vi "update driveble paths (point input).vi"(7 "possible wheel angles":i8[](array[numeric])=[-35, -30, -25, -20, -15, -10, -5, -1, 1, 5, 10, 15, 20, 25, 30, 35], 8 "y LIDAR position(in)":i16, 9 "x LIDAR position(in)":i16, 10 "max path lengths":u16[](array[numeric])=[0, 0, 0, 0, 0, 0, 0, 0, 0, 0, 0, 0, 0, 0, 0, 0], 11 "number 16\" iterations":i32) -> (2 "updated max path lengths":u16[](array[numeric]))   [LabVIEW 2009]
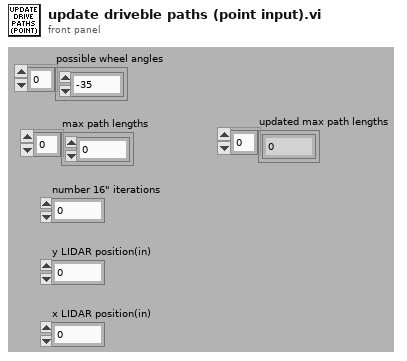
[diagram p1: front panel]
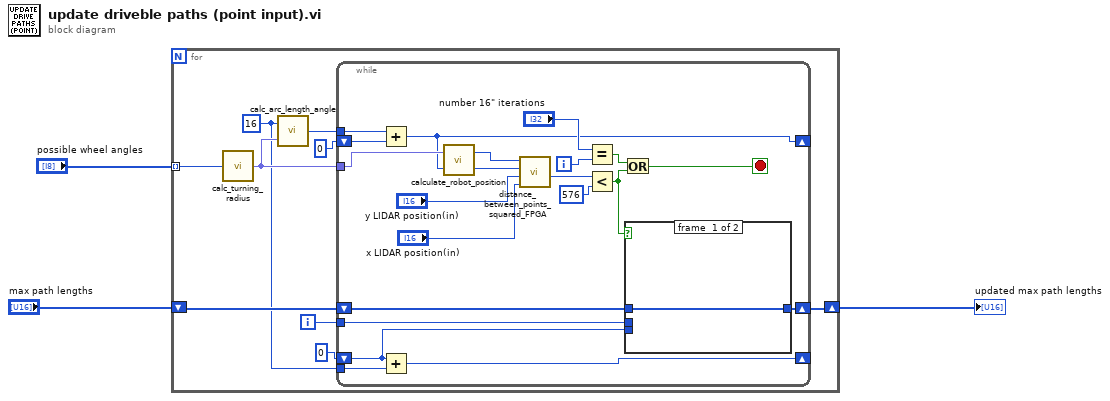
[diagram p0: block diagram]
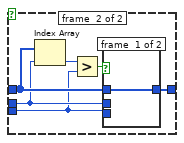
[diagram p2: hidden frame]
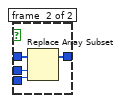
[diagram p3: hidden frame]
diagram:
  n1 = for {
    tunnel: "possible wheel angles" -> [w4] mode=indexing
    shift-right: [w7] -> w1
    shift-left: "max path lengths" -> [w9]
    i -> [w8]
    w6 = u16 16 ("Distance Along Arc")
    n2 = call "calc_turning_radius.vi"("Wheel Angle"=w4) -> ("Turning Radius (in)"=w12:fxp<+/-,22,12>)
    n3 = call "calc_arc_length_angle.vi"("Turning Radius (in)"=w12, "Distance Along Arc"=w6) -> ("arc length angle"=w11:u16)
    n4 = while {
      tunnel: w12 -> [w32]
      tunnel: w11 -> [w33]
      shift-right: [w16] -> _
      shift-left: u16 0 ("arc length angle") -> [w24]
      tunnel: w8 -> [w23]
      shift-right: [w22] -> w7
      shift-left: w9 -> [w25]
      tunnel: w6 -> [w15]
      shift-right: [w14] -> _
      shift-left: u16 0 -> [w13]
      i -> [w21]
      stop <- w17 stop-if-true
      n5 = Add(x=w33, y=w24) -> (x+y=w16:u16)
      n6 = Add(x=w13, y=w15) -> (x+y=w14:u16)
      n7 = call "calculate_robot_position.vi"("arc length angle"=w16, "Turning Radius (in)"=w32) -> ("New Y Position"=w30:i16, "New X Position"=w31:i16)
      n8 = call "distance_between_points_squared_FPGA.vi"("x LIDAR position"="x LIDAR position(in)", "y LIDAR position"="y LIDAR position(in)", "y position"=w30, "x position"=w31) -> ("distance squared"=w27:i32)  [unwired: 7 in]
      n9 = Equal?(x="number 16\" iterations", y=w21) -> (x = y?=w18:bool)
      n10 = Less?(x=w27, y=576) -> (x < y?=w19:bool)
      n11 = Or(x=w18, y=w19) -> (x .or. y?=w17:bool)
      n12 = case shown="True" w19 {
        tunnel: w25 -> [w34 w39]
        tunnel: w13 -> [_ w36]
        tunnel: w23 -> [_ w38]
        tunnel: [w34 w40] -> w22
        frame #0 {
        }
        frame #1 {
          n13 = Index Array(array=w39, index=w38) -> (element=w37:u16)
          n14 = Greater?(x=w37, y=w36) -> (0:w35:bool)
          n15 = case shown="False" w35 {
            tunnel: [w41 w45] -> w40
            tunnel: w39 -> [w41 w44]
            tunnel: w38 -> [_ w43]
            tunnel: w36 -> [_ w42]
            frame #0 {
            }
            frame #1 {
              n16 = Replace Array Subset(array=w44, new element=w42, index=w43) -> (w45:u16[])
            }
          }
        }
      }
    }
  }
  "updated max path lengths" <- w1
